vi "AccumulateHistogram.vi"(8 "Array in":i32[](array[numeric]), 11 "Histogram graph in":T1) -> (0 "Array out":i32[](array[numeric]), 3 "Histogram graph out":T1)   [LabVIEW 2011]
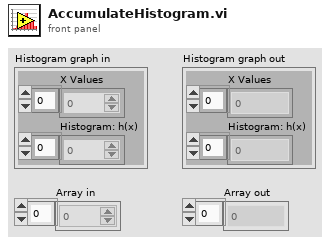
[diagram p1: front panel]
types:
  T1 = cluster{"X Values":dbl[], "Histogram: h(x)":i32[]}
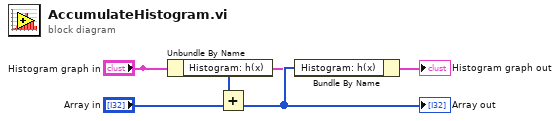
[diagram p0: block diagram]
diagram:
  n1 = Unbundle By Name("Histogram graph in") -> ("Histogram: h(x)"=w4:i32[])
  n2 = Add(x=w4, y="Array in") -> (x+y=w5:i32[])
  "Array out" <- w5
  n3 = Bundle By Name(cluster="Histogram graph in", "Histogram: h(x)"=w5) -> (→"Histogram graph out":T1)
